vi "Element Init.vi"(7 "VolatusAPI":refnum<class "VolatusAPI.lvclass">, 8 "error in (no error)":errorcluster, 10 "JSON":string, 11 "DblNumericStatusIndicator in":refnum<class "DblStatusIndicator.lvclass">) -> (0 "error out":errorcluster, 3 "DblNumericStatusIndicator out":refnum<class "DblStatusIndicator.lvclass">)   [LabVIEW 2020, in "VolatusGUIElements.lvlib" / "DblStatusIndicator.lvclass"]
uses:
  DblStatusIndicator.lvclass
  C:/dev/lv20CE/relink/lv-volatus/VolatusGUI/GUI Element/GUI Element.lvclass
  Volatus/VolatusAPI/VolatusAPI.lvclass
  JSON.ctl
  lv-vecto/Vecto/Group DBL/Group DBL.lvclass
  C:/dev/lv20CE/relink/lv-vecto/Vecto/Group/Group.lvclass
  VolatusGUI/GUI Element/GUI Element.lvclass/GUI Element.ctl
  DblStatusIndicator.lvclass/DblStatusIndicator.ctl
  c840d708-a4aa-4e42-9474-a77b72826cb9.vi
  <vilib>/JDP Science/JSONtext/JSON text to Variant.vi
  <vilib>/JDP Science/JSONtext/LVClass Serializer/JSONtext LVClass Serializer.lvclass
  VolatusGUI/GUI Element/GUI Element.lvclass
  VolatusGUIElements.lvlib
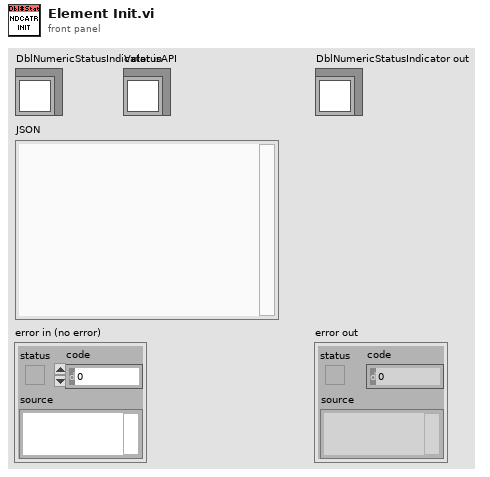
[diagram p1: front panel]
types:
  T1 = typedef "VolatusGUIElements.lvlib/DblStatusIndicator.lvclass/JSON.ctl" = cluster{"Channel":string, "Staleness":dbl, "Format":string, "Color":string}
  T2 = typedef "VectoConfig.lvlib/Channel Info.ctl" = cluster{"Name":string, "Group":string, "Owning Node":string, "Owning Task":string, "Resource":string}
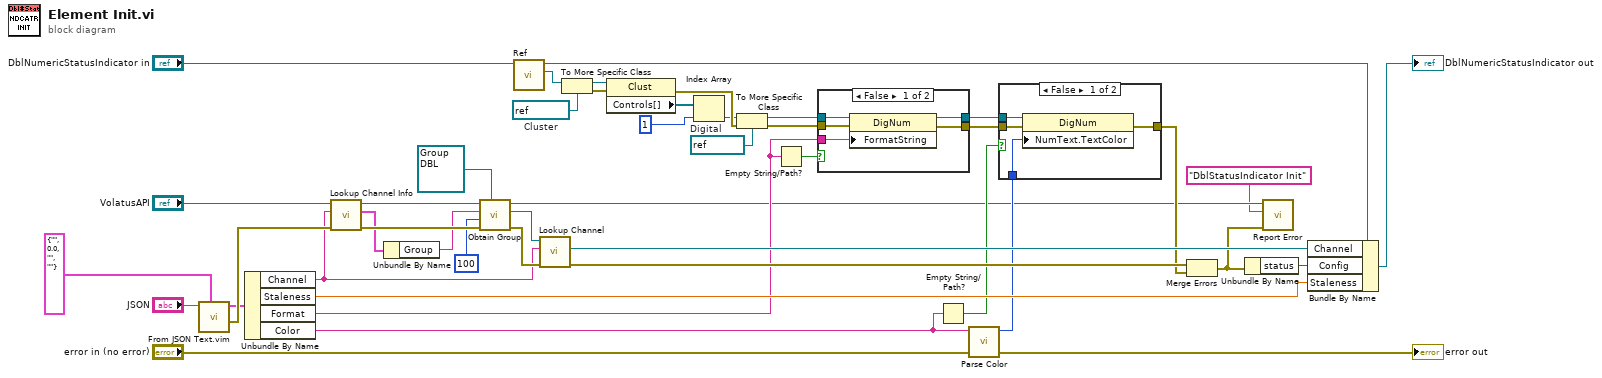
[diagram p0: block diagram]
diagram:
  w22 = refnum<vi> refnum  # Digital
  w26 = refnum<vi> refnum  # Cluster
  n1 = call "From JSON Text.vim"("Data Type and Default Value"=T1 {"Channel"="", "Staleness"=0.0, "Format"="", "Color"=""} ("JSON"), "JSON"="JSON") -> ("error out"=w44:errorcluster, "Data out"=w40:T1)  [unwired: 8 in]
  n2 = Unbundle By Name(w40) -> ("Channel"=w15:string, "Staleness"=w34:dbl, "Format"=w12:string, "Color"=w6:string)
  n3 = call "Lookup Channel Info.vi"("error in (no error)"=w44, "Channel Name"=w15, "VolatusAPI in"="VolatusAPI") -> ("error out"=w16:errorcluster, "Channel Info"=w14:T2, "VolatusAPI out"=w17:refnum<class "VolatusAPI.lvclass">)  [unwired: 5 in, 1 out]
  n4 = Unbundle By Name(w14) -> ("Group"=w13:string)
  n5 = call "Obtain Group.vi"("Group Type (Abstract)"=refnum<class "Group DBL.lvclass"> refnum ("Group in"), "error in (no error)"=w16, "Timeout ms (5000)"=u32 100, "Group Name"=w13, "VolatusAPI in"=w17) -> ("error out"=w39:errorcluster, "Group"=w36:refnum<class "Group DBL.lvclass">, "VolatusAPI out"=w4:refnum<class "VolatusAPI.lvclass">)  [unwired: 4 in]
  n6 = call "Ref.vi"("GUI Element in"="DblNumericStatusIndicator in") -> ("Ref"=w27:refnum<vi>, "GUI Element out"=w29:refnum<class "DblStatusIndicator.lvclass">)  [unwired: 9 in]
  n7 = call "Lookup Channel.vi"("error in (no error)"=w39, "Channel Name"=w15, "Group in"=w36) -> ("error out"=w25:errorcluster, "Channel"=w38:refnum<class "Channel DBL.lvclass">)  [unwired: 6 in, 1 out]
  n8 = To More Specific Class(target class=w26, reference=w27) -> (specific class reference=w28:refnum<vi>, error out=w19:errorcluster)  [unwired: 1 in]
  n9 = property class="Clust"(reference=w28, error in=w19) -> (error out=w43:errorcluster, "Controls[]"=w24:refnum<vi>[])  [unwired: 1 out]
  n10 = Index Array(array=w24, index=1) -> (element=w23:refnum<vi>)
  n11 = To More Specific Class(target class=w22, reference=w23, error in=w43) -> (specific class reference=w21:refnum<vi>, error out=w20:errorcluster)
  n12 = Empty String/Path?(string/path=w12) -> (empty?=w11:bool)
  n13 = case shown="False" w11 {
    tunnel: w21 -> [w49 w51]
    tunnel: w20 -> [w48 w50]
    tunnel: w12 -> [w47 _]
    tunnel: [w46 w51] -> w10
    tunnel: [w45 w50] -> w9
    frame False {
      n14 = property class="DigNum"(reference=w49, error in=w48, "FormatString"=w47) -> (reference out=w46:refnum<vi>, error out=w45:errorcluster)
    }
    frame True {
    }
  }
  n15 = Empty String/Path?(string/path=w6) -> (empty?=w5:bool)
  n16 = call "Parse Color.vi"("Color String"=w6) -> ("Color"=w7:u32)  [unwired: 9 in, 1 out]
  n17 = case shown="False" w5 {
    tunnel: w10 -> [w55 _]
    tunnel: w9 -> [w54 w56]
    tunnel: [w53 w56] -> w8
    tunnel: w7 -> [w52 _]
    frame False {
      n18 = property class="DigNum"(reference=w55, error in=w54, "NumText.TextColor"=w52) -> (error out=w53:errorcluster)  [unwired: 1 out]
    }
    frame True {
    }
  }
  n19 = Merge Errors(w25, w8) -> (w3:errorcluster)
  n20 = Unbundle By Name(w3) -> ("status"=w31:bool)
  n21 = call "Report Error.vi"("error in (no error)"=w3, "Context"="DblStatusIndicator Init", "VolatusAPI in"=w4) -> ()  [unwired: 7 in, 2 out]
  n22 = Bundle By Name(cluster=w29, "Channel"=w38, "Config"=w31, "Staleness"=w34) -> (→"DblNumericStatusIndicator out":refnum<class "DblStatusIndicator.lvclass">)
  "error out" <- "error in (no error)"
